vi "DB Delect data(cmd).vi"(7 "condition":string, 8 "error in (no error)":errorcluster caption="错误输入（无错误）", 10 "table":string, 11 "Connncet State":T1) -> (0 "error out":errorcluster caption="错误输出", 2 "State":bool, 3 "Connncet State out":T1)   [LabVIEW 2014]
uses:
  <vilib>/addons/database/NI_Database_API.lvlib
  Ctr/Constr.ctl
  <vilib>/addons/database/Connection.llb/Conn ObjectReference.ctl
  Ctr/Conneect State.ctl
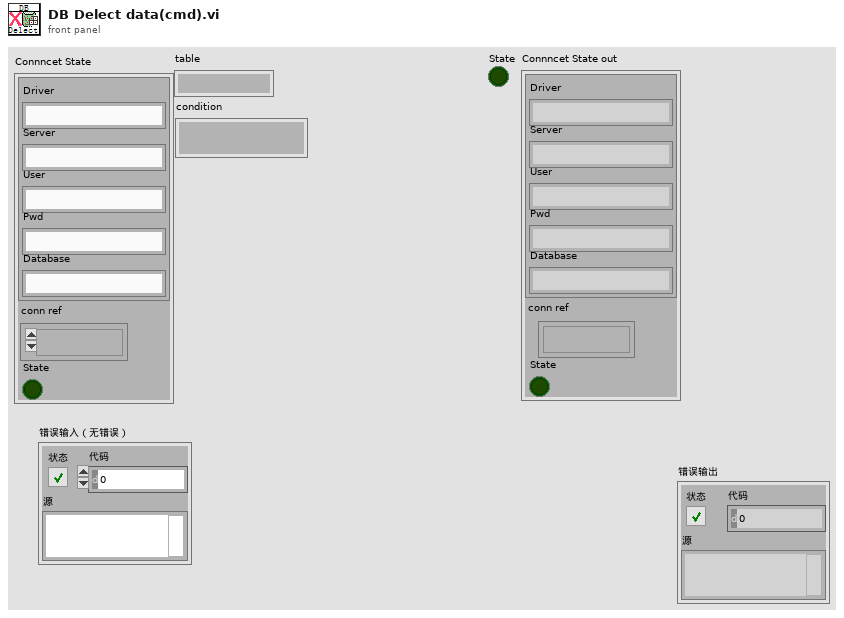
[diagram p1: front panel]
types:
  T1 = typedef "Conneect State.ctl" = cluster{"Constr":T2, "conn ref":T3, "State":bool}
  T2 = typedef "Constr.ctl" = cluster{"Driver":string, "Server":string, "User":string, "Pwd":string, "Database":string}
  T3 = typedef "NI_Database_API.lvlib/Conn ObjectReference.ctl" = refnum<k1>
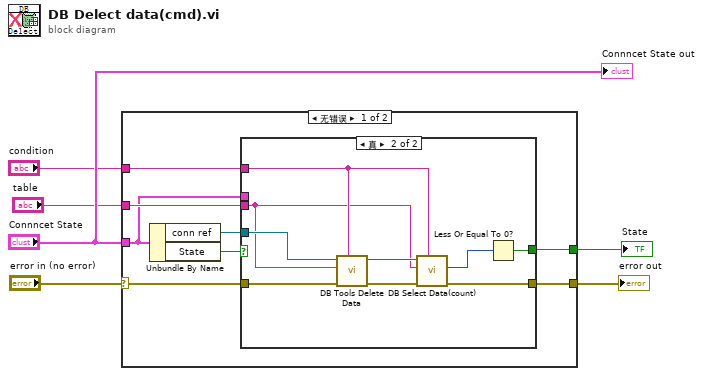
[diagram p0: block diagram]
diagram:
  n1 = case shown="无错误" "error in (no error)" {
    selector: "error in (no error)" -> [w13 w25]
    tunnel: "Connncet State" -> [w9 _]
    tunnel: "table" -> [w11 _]
    tunnel: "condition" -> [w10 _]
    tunnel: [w8 w25] -> w2
    tunnel: [w7 _] -> w1
    frame No Error {
      n2 = Unbundle By Name(w9) -> ("conn ref"=w12:T3, "State"=w14:bool)
      n3 = case shown="真" w14 {
        tunnel: w13 -> [w15 w24]
        tunnel: w12 -> [_ w23]
        tunnel: w11 -> [_ w18]
        tunnel: w10 -> [_ w19]
        tunnel: w9 -> [_ _]
        tunnel: [w15 w21] -> w8
        tunnel: [_ w17] -> w7
        frame False {
        }
        frame True {
          n4 = call <vilib>:"DB Tools Delete Data.vi"("condition"=w19, "error in (no error)"=w24, "table"=w18, "connection reference"=w23) -> ("error out"=w22:errorcluster, "connection reference out"=w20:T3)  [unwired: 6 in]
          n5 = call "DB Select Data(count).vi"("condition"=w19, "error in (no error)"=w22, "table"=w18, "connection reference"=w20) -> ("error out"=w21:errorcluster, "Count"=w16:i32)  [unwired: 5 in, 1 out]
          n6 = Less Or Equal To 0?(x=w16) -> (x <= 0?=w17:bool)
        }
      }
    }
    frame Error {
    }
  }
  "error out" <- w2
  "State" <- w1
  "Connncet State out" <- "Connncet State"
